vi "AODO-Initialize AO.vi"(0 "AO":T2, 5 "Regen?":bool, 7 "external trig":bool, 9 "AO data":dbl[][](array[numeric]), 11 "error in (no error)":errorcluster, 12 "Finite":bool) -> (4 "Tasks Out":T1[](array[typedef]), 8 "Sync Task":refnum<k21>, 10 "Start Trigger Terminal":string, 15 "error out":errorcluster)   [LabVIEW 2020]
uses:
  Typedefs/AODO-Output Spec.ctl
  Typedefs/AODO-Task Specification.ctl
panel:
  in  "Trig Src":string
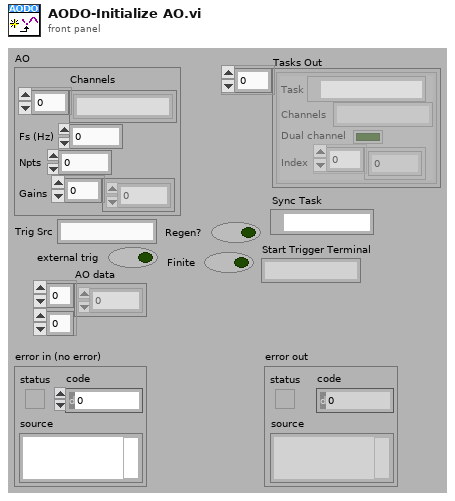
[diagram p1: front panel]
types:
  T1 = typedef "AODO-Task Specification.ctl" = cluster{"Task":refnum<k21>, "Channels":string, "Dual channel":bool, "Index":i32[]}
  T2 = typedef "AODO-Output Spec.ctl" = cluster{"Channels":string[], "Fs (Hz)":dbl, "Npts":i32, "Gains":dbl[]}
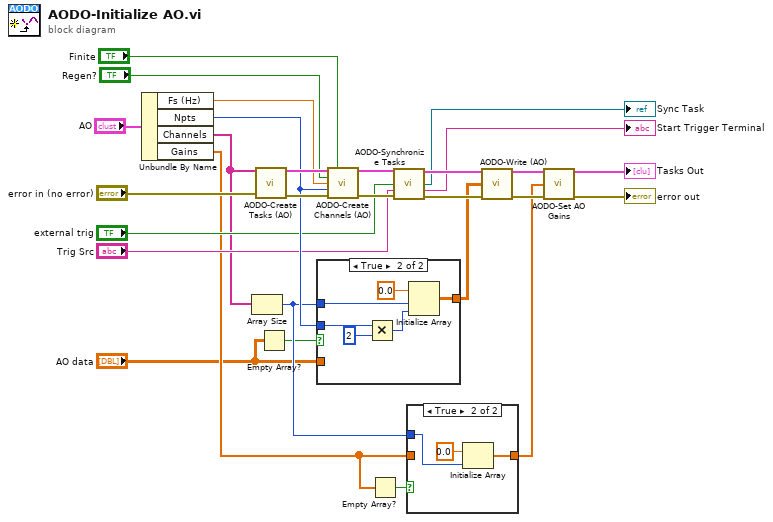
[diagram p0: block diagram]
diagram:
  n1 = Unbundle By Name("AO") -> ("Fs (Hz)"=w24:dbl, "Npts"=w19:i32, "Channels"=w6:string[], "Gains"=w8:dbl[])
  n2 = Array Size(array=w6) -> (size(s)=w10:i32)
  n3 = call "AODO-Create Tasks (AO).vi"("Channels"=w6, "error in (no error)"="error in (no error)") -> ("Task Specs"=w26:T1[], "error out"=w25:errorcluster)  [unwired: 12 in]
  n4 = Empty Array?(array="AO data") -> (empty?=w5:bool)
  n5 = case shown="True" w5 {
    tunnel: w19 -> [_ w34]
    tunnel: [w29 w32] -> w18
    tunnel: w10 -> [_ w30]
    tunnel: "AO data" -> [w29 _]
    frame False {
    }
    frame True {
      n6 = Multiply(x=w34, y=2) -> (x*y=w33:i32)
      n7 = Initialize Array(0.0 ("element"), w30, w33) -> (w32:dbl[][])
    }
  }
  n8 = call "AODO-Create Channels (AO).vi"("Tasks In"=w26, "Finite"="Finite", "Regen?"="Regen?", "Fs (Hz)"=w24, "Npts"=w19, "error in (no error)"=w25) -> ("Tasks Out"=w23:T1[], "error out"=w22:errorcluster)  [unwired: 8 in]
  n9 = Empty Array?(array=w8) -> (empty?=w9:bool)
  n10 = call "AODO-Synchronize Tasks.vi"("Tasks In"=w23, "external trig"="external trig", "Trig Src"="Trig Src", "error in (no error)"=w22) -> ("Tasks Out"=w21:T1[], "Sync Task"=→"Sync Task":refnum<k21>, "Start Trigger Terminal"=→"Start Trigger Terminal":string, "error out"=w20:errorcluster)  [unwired: 8 in]
  n11 = case shown="True" w9 {
    tunnel: w10 -> [_ w39]
    tunnel: w8 -> [w36 _]
    tunnel: [w36 w38] -> w7
    frame False {
    }
    frame True {
      n12 = Initialize Array(0.0 ("element"), w39) -> (w38:dbl[])
    }
  }
  n13 = call "AODO-Write (AO).vi"("Tasks In"=w21, "AO Waveforms"=w18, "error in (no error)"=w20) -> ("Tasks Out"=w14:T1[], "error out"=w13:errorcluster)  [unwired: 11 in]
  n14 = call "AODO-Set AO Gains.vi"("Tasks"=w14, "Gains"=w7, "error in (no error)"=w13) -> ("Tasks out"=→"Tasks Out":T1[], "error out"=→"error out":errorcluster)  [unwired: 11 in]
